vi "Interface_Implement.vi"(11 "ClassThatImplements":refnum<class>) -> (3 "InterfaceHelpClass":refnum<class>)   [LabVIEW 2010]
doc: "Implemnts an Interface"
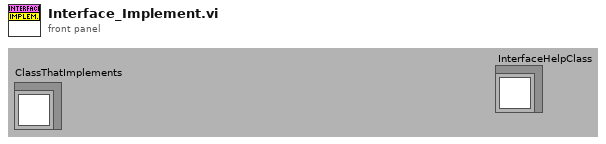
[diagram p1: front panel]
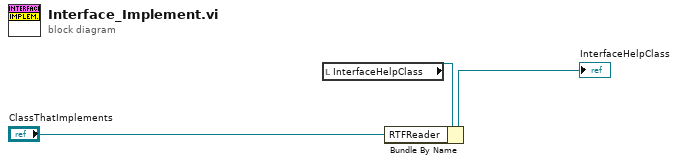
[diagram p0: block diagram]
diagram:
  n1 = local read "InterfaceHelpClass"() -> (w1:refnum<class>)
  n2 = Bundle By Name(cluster=w1, "RTFReader"="ClassThatImplements") -> (→"InterfaceHelpClass":refnum<class>)
